vi "Get_FPGASimIO_Status_5734.vi"(8 "Error In":errorcluster) -> (0 "Error Out":errorcluster, 3 "Sim IO FPGA Status":bool)   [LabVIEW 2012]
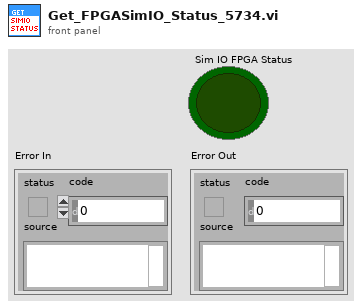
[diagram p1: front panel]
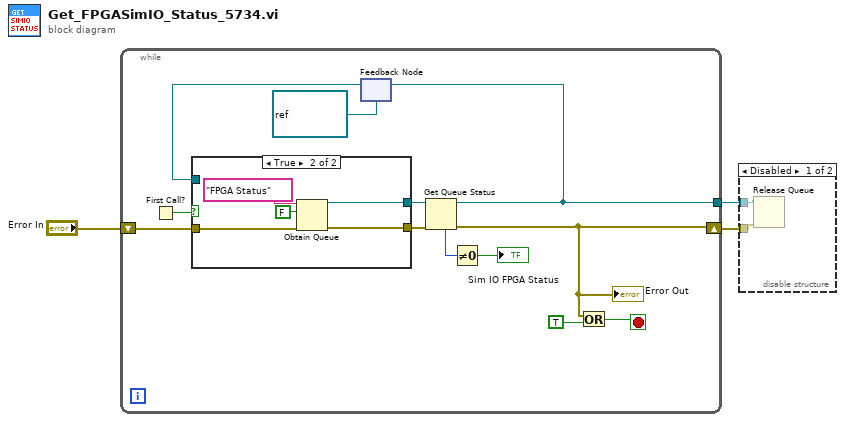
[diagram p0: block diagram]
diagram:
  n1 = while {
    shift-right: [w15] -> w3
    shift-left: "Error In" -> [w8]
    tunnel: [w7] -> w1
    stop <- w13 stop-if-true
    n2 = First Call?() -> (First Call?: T/F=w9:bool)
    n3 = feedback #1(refnum<queue> refnum ("queue out")) -> (w10:refnum<queue>)
    n4 = case shown="True" w9 {
      tunnel: [w17 w20] -> w12
      tunnel: [w16 w19] -> w11
      tunnel: w10 -> [w17 _]
      tunnel: w8 -> [w16 w18]
      frame False {
      }
      frame True {
        n5 = Obtain Queue(name (unnamed)="FPGA Status", element data type=FALSE, error in (no error)=w18) -> (queue out=w20:refnum<queue>, error out=w19:errorcluster)  [unwired: 2 in, 1 out]
      }
    }
    n6 = Get Queue Status(queue=w12, error in (no error)=w11) -> (queue out=w7:refnum<queue>, error out=w15:errorcluster, # elements in queue=w5:i32)  [unwired: 1 in, 5 out]
    "Error Out" <- w15
    n7 = feedback-in #1(w7) -> ()
    n8 = Not Equal To 0?(x=w5) -> (x != 0?=→"Sim IO FPGA Status":bool)
    n9 = Or(x=w15, y=TRUE ("stop")) -> (x .or. y?=w13:bool)
  }
  n10 = disable-structure shown="Disabled" {
    disable-tunnel: w3 -> [w24 _]
    disable-tunnel: w1 -> [w23 _]
    frame Disabled {
      n11 = Release Queue(queue=w23, error in (no error)=w24) -> ()  [unwired: 1 in, 3 out]
    }
    frame Enabled {
    }
  }
